vi "SetFunctionClass.vi"(8 "error in (no error)":errorcluster, 10 "FunctionClass":variant, 11 "PmuAnalysis in":refnum<class "PmuAnalysis.lvclass">) -> (0 "error out":errorcluster, 3 "PmuAnalysis out":refnum<class "PmuAnalysis.lvclass">)   [LabVIEW 2018, in "AnalysisPlugins.lvlib" / "PmuAnalysis.lvclass"]
uses:
  PmuAnalysis.lvclass
  PmuAnalysis.lvclass/PmuAnalysis.ctl
  Accessors/Read Function.vi
  Accessors/Write Function.vi
  FGen/MemberClasses/FunctionBaseClass/FunctionBase.lvclass
panel:
  # "Not all analysis plugins will\nhave function classes"
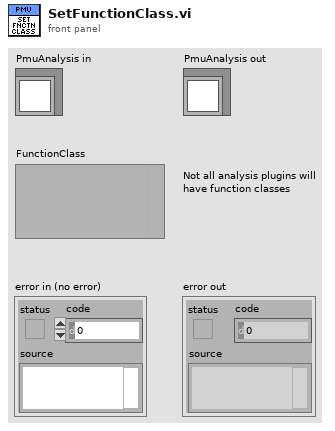
[diagram p1: front panel]
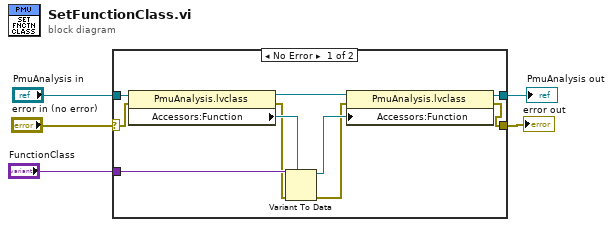
[diagram p0: block diagram]
diagram:
  n1 = case shown="No Error" "error in (no error)" {
    selector: "error in (no error)" -> [w9 w16]
    tunnel: "PmuAnalysis in" -> [w15 w17]
    tunnel: "FunctionClass" -> [w11 _]
    tunnel: [w6 w16] -> w1
    tunnel: [w10 w17] -> w2
    frame No Error {
      n2 = property class="PmuAnalysis.lvclass"(reference=w15, error in=w9) -> (reference out=w13:refnum<class "PmuAnalysis.lvclass">, error out=w8:errorcluster, "Accessors:Function"=w14:refnum<class "FunctionBase.lvclass">)
      n3 = Variant To Data(error in=w8, type=w14, Variant=w11) -> (data=w12:refnum<class "FunctionBase.lvclass">, error out=w7:errorcluster)
      n4 = property class="PmuAnalysis.lvclass"(reference=w13, error in=w7, "Accessors:Function"=w12) -> (reference out=w10:refnum<class "PmuAnalysis.lvclass">, error out=w6:errorcluster)
    }
    frame Error {
    }
  }
  "error out" <- w1
  "PmuAnalysis out" <- w2
